vi "String Boxing.vi"(8 "String After":string, 10 "Full Input String":string, 11 "String Before":string) -> (1 "String Remainder":string, 2 "String Value":string)   [LabVIEW 2012]
uses:
  <userlib>/_OpenG.lib/string/string.llb/Trim Whitespace (String)__ogtk.vi
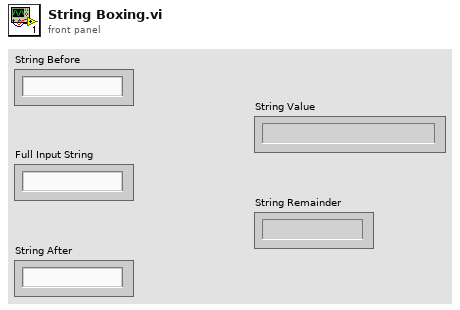
[diagram p1: front panel]
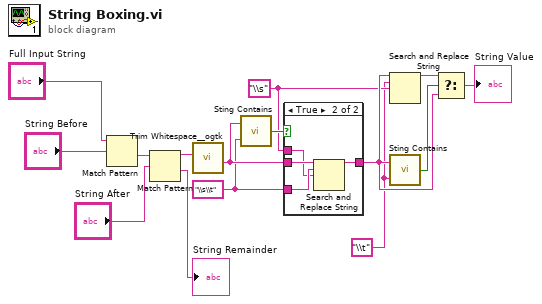
[diagram p0: block diagram]
diagram:
  w3 = "\\s" ("replace string (\"\")")
  w2 = "\\t" ("Expression to evaluate")
  w7 = "\\s\\t" ("Expression to evaluate")
  n1 = Match Pattern(string="Full Input String", regular expression="String Before") -> (after substring=w13:string)  [unwired: 1 in, 3 out]
  n2 = Match Pattern(string=w13, regular expression="String After") -> (before substring=w10:string, after substring=→"String Remainder":string)  [unwired: 1 in, 2 out]
  n3 = call-poly <userlib>:"Trim Whitespace__ogtk.vi"("String in"=w10) -> ("String out"=w8:string)  [unwired: 6 in]
  n4 = call "Sting Contains.vi"("Expression to evaluate"=w7, "Input String"=w8) -> ("Boolean"=w9:bool)
  n5 = case shown="True" w9 {
    tunnel: w8 -> [w16 w20]
    tunnel: w7 -> [_ w19]
    tunnel: [w16 w18] -> w4
    tunnel: w3 -> [_ w17]
    frame False {
    }
    frame True {
      n6 = Search and Replace String(input string=w20, search string=w19, replace string=w17) -> (result string=w18:string)  [unwired: 5 in, 3 out]
    }
  }
  n7 = Search and Replace String(input string=w4, search string=w2, replace string=w3) -> (result string=w1:string)  [unwired: 5 in, 3 out]
  n8 = call "Sting Contains.vi"("Expression to evaluate"=w2, "Input String"=w4) -> ("Boolean"=w6:bool)
  n9 = Select(t=w1, s=w6, f=w4) -> (s? t:f=→"String Value":string)
